vi "Initialize Digital Module.vi"(7 "Direction":enum16{"Input", "Output"}(ring), 8 "error in (no error)":errorcluster, 9 "Speed":enum16{"High Speed", "Low Speed"}(ring), 10 "Channels":u8, 11 "Module in":refnum<class "Module.lvclass">) -> (0 "error out":errorcluster, 3 "Module out":refnum<class "Module.lvclass">)   [LabVIEW 2015, in "Module.lvclass"]
uses:
  Module.lvclass
  Module Configuration.ctl
  Module.lvclass/Module.ctl
  VI/Module Loop/Module Loop.lvclass
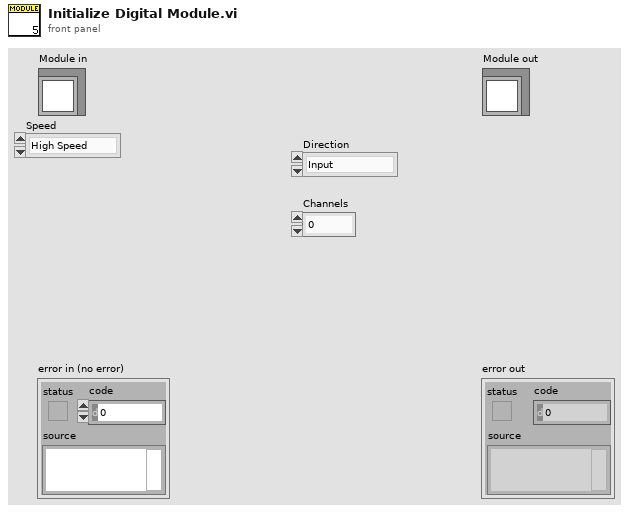
[diagram p1: front panel]
types:
  T1 = typedef "Module Loop.lvclass/Module Configuration.ctl" = cluster{"Type":string, "Direction":string, "Speed":string, "Channels":string, "FXP Type":string}
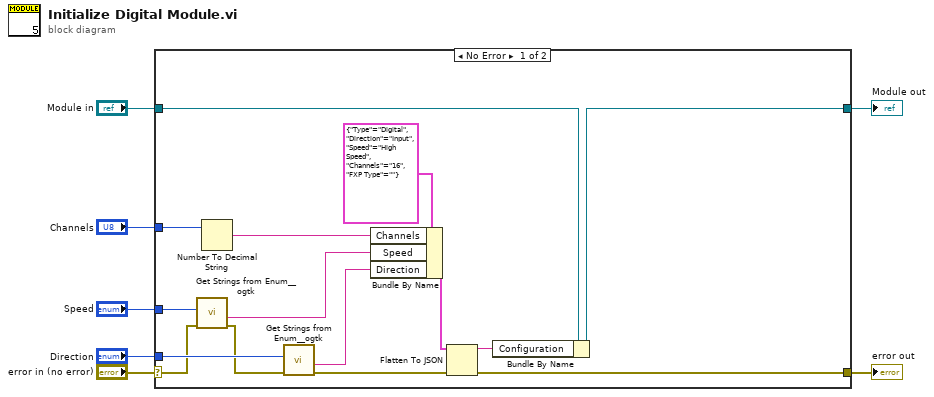
[diagram p0: block diagram]
diagram:
  n1 = case shown="No Error" "error in (no error)" {
    selector: "error in (no error)" -> [w11 w24]
    tunnel: [w16 w24] -> w6
    tunnel: [w12 w23] -> w4
    tunnel: "Module in" -> [w13 w23]
    tunnel: "Direction" -> [w22 _]
    tunnel: "Channels" -> [w19 _]
    tunnel: "Speed" -> [w9 _]
    frame No Error {
      n2 = call <userlib>:"Get Strings from Enum__ogtk.vi"("error in (no error)"=w11, "Enum"=w9) -> ("error out"=w10:errorcluster, "String Value"=w8:string)  [unwired: 6 in, 2 out]
      n3 = Number To Decimal String(number=w19) -> (decimal integer string=w18:string)  [unwired: 1 in]
      n4 = call <userlib>:"Get Strings from Enum__ogtk.vi"("error in (no error)"=w10, "Enum"=w22) -> ("error out"=w17:errorcluster, "String Value"=w20:string)  [unwired: 6 in, 2 out]
      n5 = Bundle By Name(cluster=T1 {"Type"="Digital", "Direction"="Input", "Speed"="High Speed", "Channels"="16", "FXP Type"=""} ("Cluster"), "Channels"=w18, "Speed"=w8, "Direction"=w20) -> (w15:T1)
      n6 = Flatten To JSON(anything=w15, error in (no error)=w17) -> (JSON string=w14:string, 11:w16:errorcluster)  [unwired: 1 in]
      n7 = Bundle By Name(cluster=w13, "Configuration"=w14) -> (w12:refnum<class "Module.lvclass">)
    }
    frame Error {
    }
  }
  "error out" <- w6
  "Module out" <- w4
